vi "Prompt for Step--Init UI.vi"(8 "error in (no error)":errorcluster, 10 "Control Ref Map":map{string, refnum<vi>}(c390), 11 "Keyboard Action in":refnum<class "Keyboard Action.lvclass">) -> (0 "error out":errorcluster, 3 "Keyboard Action out":refnum<class "Keyboard Action.lvclass">)   [LabVIEW 2020, in "MacroAssert.lvlib" / "Keyboard Action.lvclass"]
doc: "Initializes the user interface within the \"Prompt for Step\" VI."
uses:
  Keyboard Action.lvclass
  C:/Users/User/Documents/LabVIEW Data/Projects/MacroAssert/source/Classes/Step/Step.lvclass
  4524efd6-7cb2-439c-a68f-8d932fed4b52.vi
  Support/Get Control Reference by Label (1D STR).vi
  <vilib>/Utility/error.llb/Error Cluster From Error Code.vi
  Action Step/Action Step.lvclass
  MacroAssert.lvlib
  SubVIs/Custom Errors/Custom Errors.lvlib
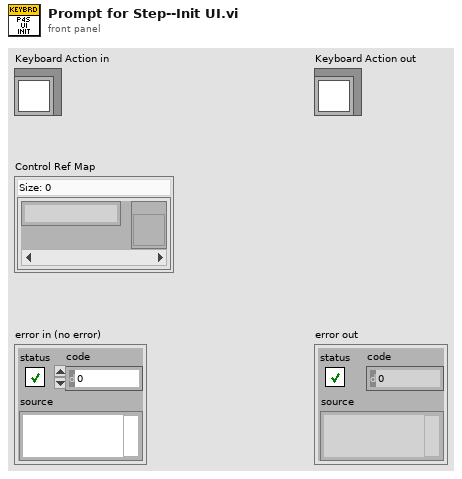
[diagram p1: front panel]
types:
  T1 = typedef "MacroAssert.lvlib/Keyboard Action.lvclass/Keyboard Action Type.ctl" = enum16{"Key Press", "Key Sequence", "Key Down", "Key Up"}
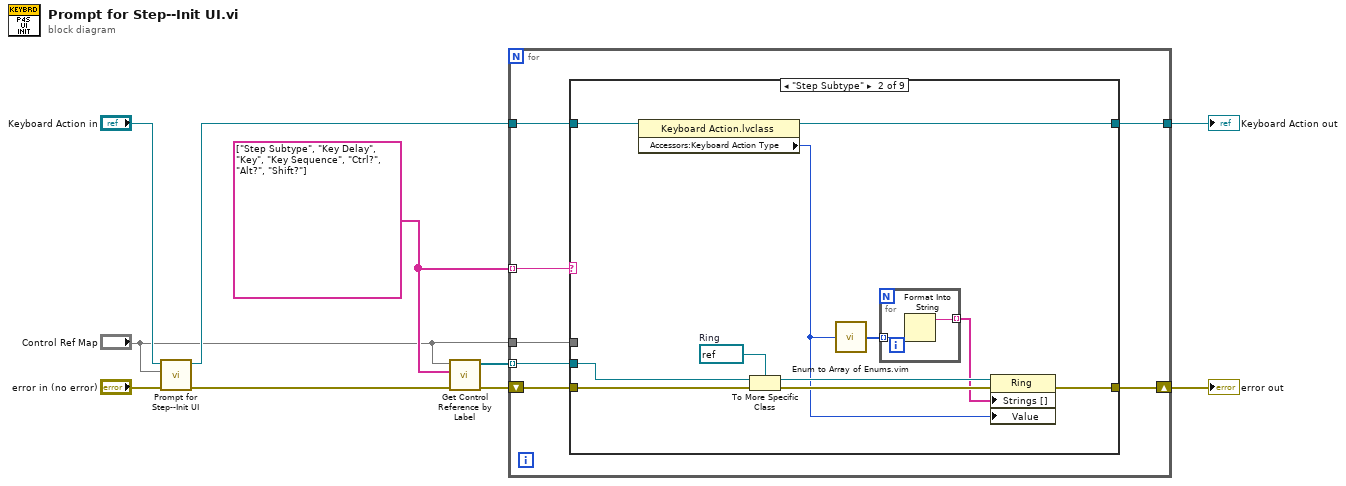
[diagram p0: block diagram]
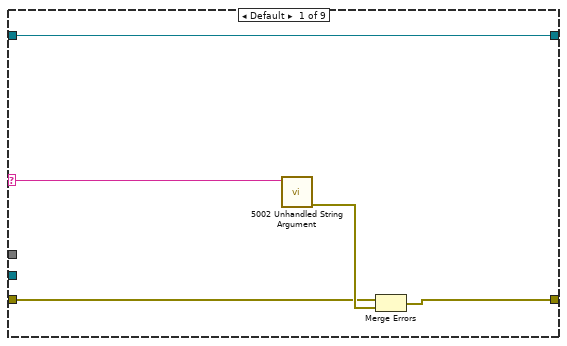
[diagram p2: hidden frame]
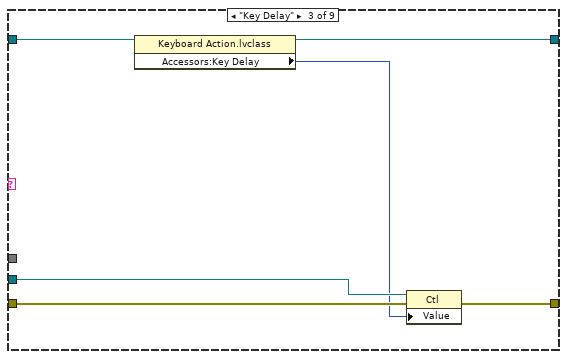
[diagram p3: hidden frame]
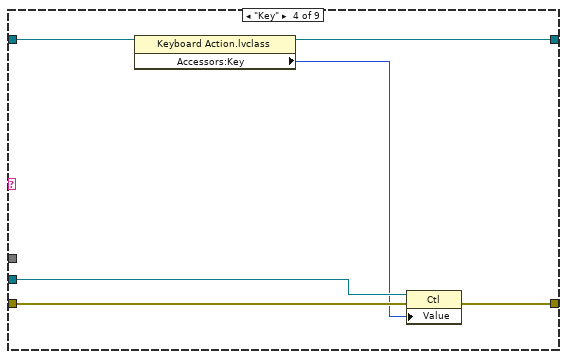
[diagram p4: hidden frame]
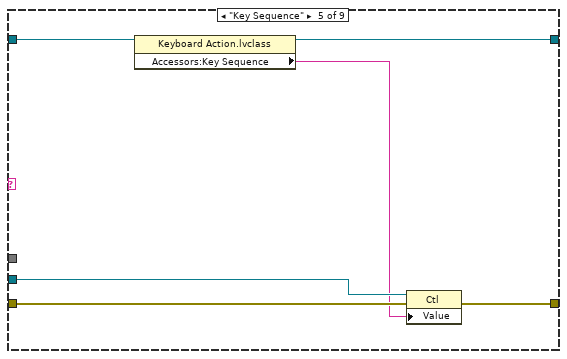
[diagram p5: hidden frame]
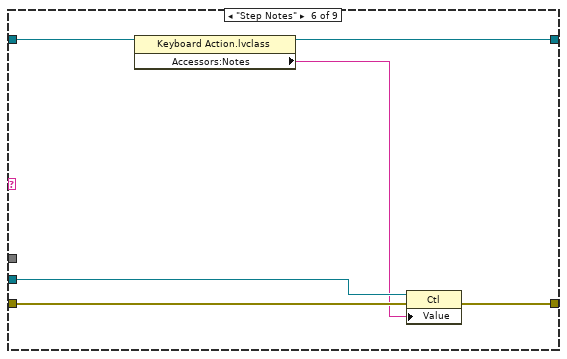
[diagram p6: hidden frame]
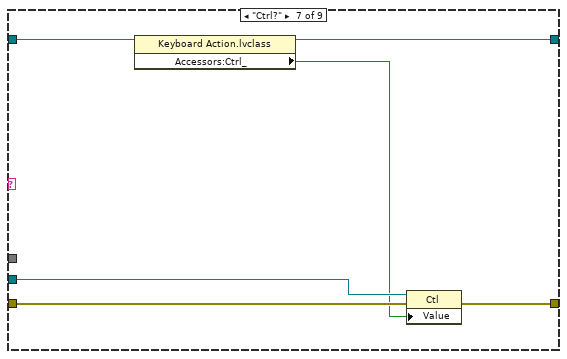
[diagram p7: hidden frame]
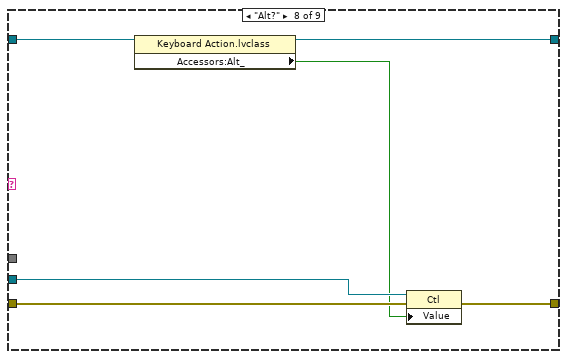
[diagram p8: hidden frame]
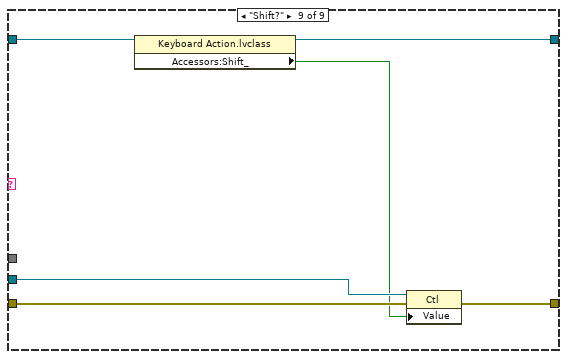
[diagram p9: hidden frame]
diagram:
  w9 = string[] ["Step Subtype", "Key Delay", "Key", "Key Sequence", "Ctrl?", "Alt?", "Shift?"]
  n1 = call-parent "Prompt for Step--Init UI.vi"("error in (no error)"="error in (no error)", "Control Ref Map"="Control Ref Map", "Step in"="Keyboard Action in") -> ("error out"=w4:errorcluster, "Step out"=w2:refnum<class "Keyboard Action.lvclass">)  [unwired: 7 in]
  n2 = call-poly "Get Control Reference by Label.vi"("error in (no error)"=w4, "Control Names"=w9, "Control Ref Map"="Control Ref Map") -> ("error out"=w10:errorcluster, "Control Refs"=w8:refnum<vi>[])  [unwired: 6 in, 1 out]
  n3 = for {
    tunnel: w2 -> [w15]
    tunnel: [w13] -> w5
    tunnel: w9 -> [w16] mode=indexing
    tunnel: w8 -> [w14] mode=indexing
    shift-right: [w12] -> w7
    shift-left: w10 -> [w17]
    tunnel: "Control Ref Map" -> [w11]
    n4 = case shown="\"Step Subtype\"" w16 {
      selector: w16 -> [w19 _ _ _ _ _ _ _ _]
      tunnel: w17 -> [w21 w27 w38 w44 w50 w56 w62 w68 w74]
      tunnel: w15 -> [w18 w26 w41 w47 w53 w59 w65 w71 w77]
      tunnel: w14 -> [_ w23 w39 w45 w51 w57 w63 w69 w75]
      tunnel: [w18 w25 w40 w46 w52 w58 w64 w70 w76] -> w13
      tunnel: [w20 w24 w36 w42 w48 w54 w60 w66 w72] -> w12
      tunnel: w11 -> [_ _ _ _ _ _ _ _ _]
      frame Default {
        n5 = call "5002 Unhandled String Argument.vi"("Argument"=w19) -> ("error out"=w22:errorcluster)  [unwired: 10 in]
        n6 = Merge Errors(w21, w22) -> (w20:errorcluster)
      }
      frame "Step Subtype" {
        w30 = refnum<vi> refnum  # Ring
        n7 = property class="Keyboard Action.lvclass"(reference=w26) -> (reference out=w25:refnum<class "Keyboard Action.lvclass">, "Accessors:Keyboard Action Type"=w29:T1)  [unwired: 1 in, 1 out]
        n8 = To More Specific Class(target class=w30, reference=w23, error in=w27) -> (specific class reference=w33:refnum<vi>, error out=w31:errorcluster)
        n9 = call "Enum to Array of Enums.vim"("enum"=w29) -> ("array of enums"=w32:T1[])
        n10 = for {
          tunnel: w32 -> [w35] mode=indexing
          tunnel: [w34] -> w28 mode=indexing
          n11 = Format Into String(w35) -> (resulting string=w34:string)  [unwired: 3 in, 1 out]
        }
        n12 = property class="Ring"(reference=w33, error in=w31, "Strings []"=w28, "Value"=w29) -> (error out=w24:errorcluster)  [unwired: 1 out]
      }
      frame "Key Delay" {
        n13 = property class="Keyboard Action.lvclass"(reference=w41) -> (reference out=w40:refnum<class "Keyboard Action.lvclass">, "Accessors:Key Delay"=w37:i32)  [unwired: 1 in, 1 out]
        n14 = property class="Ctl"(reference=w39, error in=w38, "Value"=w37) -> (error out=w36:errorcluster)  [unwired: 1 out]
      }
      frame "Key" {
        n15 = property class="Keyboard Action.lvclass"(reference=w47) -> (reference out=w46:refnum<class "Keyboard Action.lvclass">, "Accessors:Key"=w43:u8)  [unwired: 1 in, 1 out]
        n16 = property class="Ctl"(reference=w45, error in=w44, "Value"=w43) -> (error out=w42:errorcluster)  [unwired: 1 out]
      }
      frame "Key Sequence" {
        n17 = property class="Keyboard Action.lvclass"(reference=w53) -> (reference out=w52:refnum<class "Keyboard Action.lvclass">, "Accessors:Key Sequence"=w49:string)  [unwired: 1 in, 1 out]
        n18 = property class="Ctl"(reference=w51, error in=w50, "Value"=w49) -> (error out=w48:errorcluster)  [unwired: 1 out]
      }
      frame "Step Notes" {
        n19 = property class="Keyboard Action.lvclass"(reference=w59) -> (reference out=w58:refnum<class "Keyboard Action.lvclass">, "Accessors:Notes"=w55:string)  [unwired: 1 in, 1 out]
        n20 = property class="Ctl"(reference=w57, error in=w56, "Value"=w55) -> (error out=w54:errorcluster)  [unwired: 1 out]
      }
      frame "Ctrl?" {
        n21 = property class="Keyboard Action.lvclass"(reference=w65) -> (reference out=w64:refnum<class "Keyboard Action.lvclass">, "Accessors:Ctrl_"=w61:bool)  [unwired: 1 in, 1 out]
        n22 = property class="Ctl"(reference=w63, error in=w62, "Value"=w61) -> (error out=w60:errorcluster)  [unwired: 1 out]
      }
      frame "Alt?" {
        n23 = property class="Keyboard Action.lvclass"(reference=w71) -> (reference out=w70:refnum<class "Keyboard Action.lvclass">, "Accessors:Alt_"=w67:bool)  [unwired: 1 in, 1 out]
        n24 = property class="Ctl"(reference=w69, error in=w68, "Value"=w67) -> (error out=w66:errorcluster)  [unwired: 1 out]
      }
      frame "Shift?" {
        n25 = property class="Keyboard Action.lvclass"(reference=w77) -> (reference out=w76:refnum<class "Keyboard Action.lvclass">, "Accessors:Shift_"=w73:bool)  [unwired: 1 in, 1 out]
        n26 = property class="Ctl"(reference=w75, error in=w74, "Value"=w73) -> (error out=w72:errorcluster)  [unwired: 1 out]
      }
    }
  }
  "error out" <- w7
  "Keyboard Action out" <- w5
